vi "Send Configure TrigLevel.vi"(7 "Message Priority (Normal)":T1=enum."Normal", 8 "error in (no error)":errorcluster, 10 "TrigLvl":dbl[unit], 11 "Message Enqueuer":refnum<class "Message Enqueuer.lvclass">) -> (0 "error out":errorcluster, 3 "Message Enqueuer out":refnum<class "Message Enqueuer.lvclass">)   [LabVIEW 2016, in "CS++MCS.lvlib" / "Configure TrigLevel Msg.lvclass"]
doc: "Sends the <B>CS++MCS.lvlib:Configure TrigLevel Msg.lvclass</B> message.\n\n<B>CS++MCS.lvlib:CS++MCS.lvclass:Configure TrigLevel.vi</B> Description:\n\nThis VI configures the Trigger level used for analog triggering of the MCS."
uses:
  Configure TrigLevel Msg.lvclass
  <vilib>/ActorFramework/Message Enqueuer/Message Enqueuer.lvclass
  <vilib>/ActorFramework/Message Enqueuer/Message Priority.ctl
  C:/Program Files (x86)/National Instruments/LabVIEW 2016/vi.lib/ActorFramework/Message/Message.lvclass
  Configure TrigLevel Msg.lvclass/Configure TrigLevel Msg.ctl
  <vilib>/ActorFramework/Message Enqueuer/Message Enqueuer.lvclass/Message Enqueuer.ctl
  <vilib>/ActorFramework/Message Priority Queue/Priority Enqueue.vi
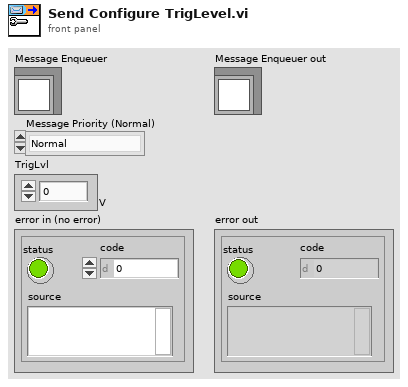
[diagram p1: front panel]
types:
  T1 = typedef "Actor Framework.lvlib/Message Enqueuer.lvclass/Message Priority.ctl" = enum16{"Low", "Normal", "High"}
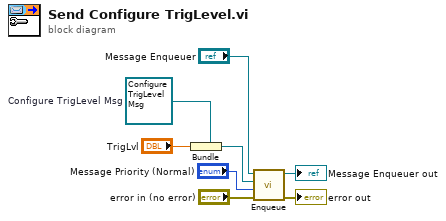
[diagram p0: block diagram]
diagram:
  w2 = refnum<class "Configure TrigLevel Msg.lvclass"> refnum  # Configure TrigLevel Msg
  n1 = Bundle(cluster=w2, "TrigLvl") -> (w5:refnum<class "Configure TrigLevel Msg.lvclass">)
  n2 = call <vilib>:"Enqueue.vi"("error in (no error)"="error in (no error)", "Message Priority (Normal)"="Message Priority (Normal)", "Message"=w5, "Message Enqueuer in"="Message Enqueuer") -> ("error out"=→"error out":errorcluster, "Message Enqueuer out"=→"Message Enqueuer out":refnum<class "Message Enqueuer.lvclass">)  [unwired: 6 in]
